vi "OE1022_Configure Harmonic.vi"(7 "OE1022_Configure Harmonic":cluster{"Harmonic 1":u16, "Harmonic 2":u16}={"Harmonic 1"=1, "Harmonic 2"=1} {"Harmonic 2" min=1 max=32767; "Harmonic 1" min=1 max=32767}, 8 "Error in (no error)":errorcluster caption="error out（no error）", 9 "Remote Mode":u16(ring) items=["USB"=0, "GPIB"=2], 11 "VISA resource name":refnum<visa-resource-name>) -> (0 "Error out":errorcluster caption="error out", 1 "Output String":string, 3 "VISA resource  out":refnum<visa-resource-name>)   [LabVIEW 2011]
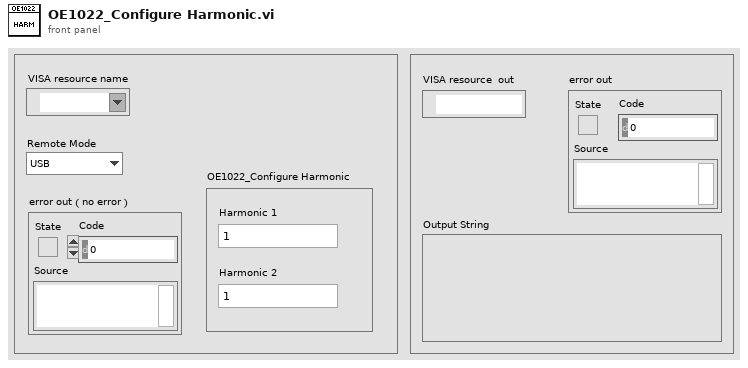
[diagram p1: front panel]
types:
  T1 = enum16{"ISRC", "IGND", "ICPL", "ILIN", "PHAS", "FMOD", "RSLP", "FREQ", "SWPT", "SLLM", "SULM", "SSLL", "SSLG", "STLM", "SWRM", "IRNG", "SENS", "RMOD", "OFLT", "OFSL", "SYNC", "DMOD", "HARM", "DARB", "SWVT", "SLVL", "SVLL", "SVUL", "SVSL", "SVSG", "SVTM", "SVRM", "RALL", "SNAP", "OUTP", "OAUX", "COUT", "CAUX", "COFP", "CEXP", "FPOP", "OEXP", "*IDN", "*RST", "OVLD", "INOV", "GNOV", "*PLL", "SSET", "RSET", "AGAN", "APHS", "ARSV", "ASCL", "EQCD", "EQCS", "SPED", "SRAT", "SLEN", "SSLE", "STRG", "SPRM", "STRD", "PAUS", "REST", "SPTS", "TRCA", "TEMP", "RSTU", "IHNZ", "DEQU", "SADD", "ARNG", "CSPE", "ISRCD", "IGNDD", "ICPLD", "ILIND", "PHASD", "FMODD", "RSLPD", "FREQD", "SWPTD", "SLLMD", "SULMD", "SSLLD", "SSLGD", "STLMD", "SWRMD", "SENSD", "RMODD", "OFLTD", "OFSLD", "SYNCD", "HARMD", "EQCDD", "EQCSD", "SNAPD", "OUTPD", "SWVTD", "SLVLD", "SVLLD", "SVULD", "SVSLD", "SVSGD", "SVTMD", "SVRMD", "SVDCD", "ARSVD", "AGAND", "APHSD", "ASCLD", "FPOPD", "CAUXD", "OEXPD", "SPEDD", "SRATD", "SLEND", "SSLED", "STRGD", "SPRMD", "STRDD", "PAUSD", "RESTD", "SPTSD", "TRCAD", "*IDND", "*RSTD", "INOVD", "GNOVD", "*PLLD", "SSETD", "RSETD"}
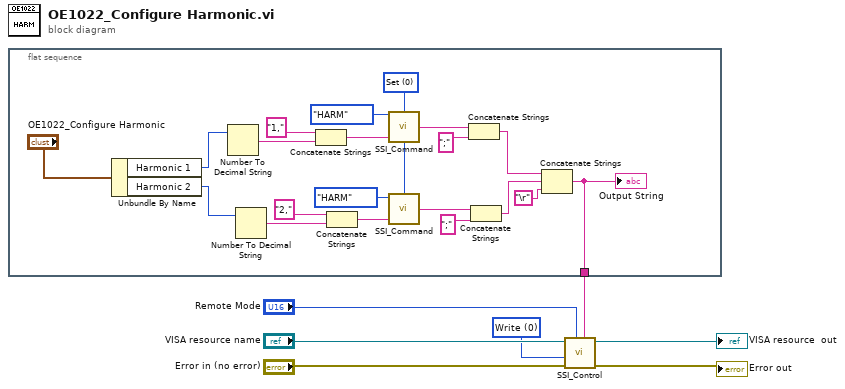
[diagram p0: block diagram]
diagram:
  w6 = u16 0 items=["Write", "Read"] ("Control")
  n1 = flat-sequence {
    tunnel: [w27] -> w1
    frame #0 {
      w21 = u16 0 items=["Set", "Query"] ("Opera")
      n2 = Unbundle By Name("OE1022_Configure Harmonic") -> ("Harmonic 1"=w25:u16, "Harmonic 2"=w20:u16)
      n3 = Number To Decimal String(number=w25) -> (decimal integer string=w13:string)  [unwired: 1 in]
      n4 = Number To Decimal String(number=w20) -> (decimal integer string=w12:string)  [unwired: 1 in]
      n5 = Concatenate Strings("1," ("字符串"), w13) -> (w9:string)
      n6 = Concatenate Strings("2," ("字符串"), w12) -> (w8:string)
      n7 = call "SSI_Command.vi"("Opera"=w21, "Paramter"=w9, "Command Type"=T1."HARM") -> ("Output string"=w15:string)  [unwired: 1 in]
      n8 = call "SSI_Command.vi"("Opera"=w21, "Paramter"=w8, "Command Type"=T1."HARM") -> ("Output string"=w14:string)  [unwired: 1 in]
      n9 = Concatenate Strings(w15, ";") -> (w17:string)
      n10 = Concatenate Strings(w14, ";") -> (w16:string)
      n11 = Concatenate Strings(w17, w16, "\r") -> (w27:string)
      "Output String" <- w27
    }
  }
  n12 = call "SSI_Control.vi"("Write Buffer"=w1, "Remote Mode"="Remote Mode", "Error in (no error)"="Error in (no error)", "Control"=w6, "VISA resource name"="VISA resource name") -> ("Error out"=→"Error out":errorcluster, "VISA resource  out"=→"VISA resource  out":refnum<visa-resource-name>)  [unwired: 3 in, 2 out]
